vi "Get DDG Lite Control Byte.vi"(8 "error in (no error)":errorcluster, 10 "control":string, 11 "channel":u32(ring)=65535 items=["AT_DDGLite_ChannelA"=1073741824, "AT_DDGLite_ChannelB"=1073741825, "AT_DDGLite_ChannelC"=1073741826]) -> (0 "error out":errorcluster, 2 "control out":string, 3 "function return":u32)   [LabVIEW 2014, in "atmcd32d.lvlib"]
doc: "unsigned int WINAPI GetDDGLiteControlByte(AT_DDGLiteChannelId channel, unsigned char * control);"
uses:
  atmcd32d.lvlib
  atmcd32d.dll
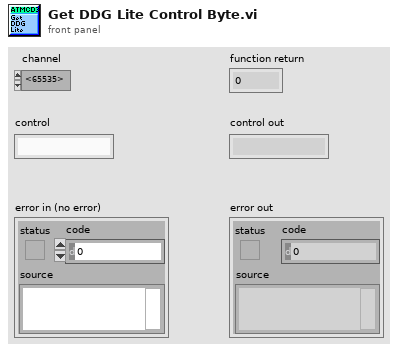
[diagram p1: front panel]
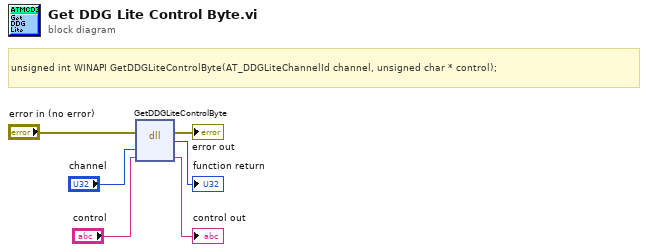
[diagram p0: block diagram]
diagram:
  # "unsigned int WINAPI GetDDGLiteControlByte(AT_DDGLiteChannelId channel, unsigned char * control);"
  n1 = dll-call lib="C:/Users/Bakir/Documents/Lambda2-Testing/lib/Andorlib/atmcd32d.*" fn="GetDDGLiteControlByte"(error in="error in (no error)", "channel"="channel", "control"="control") -> (error out=→"error out":errorcluster, →"function return":u32, "control"=→"control out":string)  [unwired: 3 in, 1 out]
